vi "Destroy.vi"(0 "reference in":refnum<class "GetCurrentInfoCommand.lvclass">, 11 "Error In":errorcluster) -> (4 "reference out":refnum<class "GetCurrentInfoCommand.lvclass">, 15 "Error Out":errorcluster)   [LabVIEW 2024, in "GetCurrentInfoCommand.lvclass"]
uses:
  GetCurrentInfoCommand.lvclass/GetCurrentInfoCommand.ctl
  GetCurrentInfoCommand.lvclass
panel:
  # "Connector Pane"
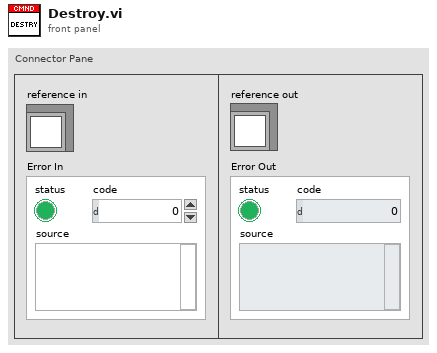
[diagram p1: front panel]
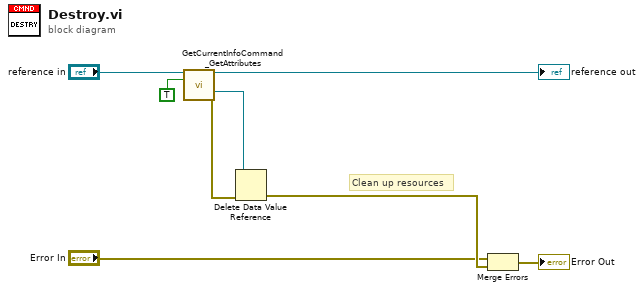
[diagram p0: block diagram]
diagram:
  # "Clean up resources"
  n1 = call "GetCurrentInfoCommand_GetAttributes.vi"("reference in"="reference in", "OnlyGetDvrReference(False)"=TRUE) -> ("reference out"=→"reference out":refnum<class "GetCurrentInfoCommand.lvclass">, "DataRef"=w4:refnum<data-value>, "Error Out"=w5:errorcluster)  [unwired: 10 in, 1 out]
  n2 = Delete Data Value Reference(data value reference=w4, error in=w5) -> (error out=w3:errorcluster)  [unwired: 1 out]
  n3 = Merge Errors("Error In", w3) -> (→"Error Out":errorcluster)
